vi "Build Item Graph from Type.vi"(9 "OwningVI":refnum<vi>, 10 "Max Depth (12)":i32=12, 11 "Type":variant) -> (0 "error out":errorcluster, 3 "Item Graph":T1[](array[typedef]))   [LabVIEW 2020, in "Better Search.lvlib"]
uses:
  Better Search.lvlib
  Data Types/Type Reflection Item.ctl
  <vilib>/Utility/Data Type/NI_Data Type.lvlib
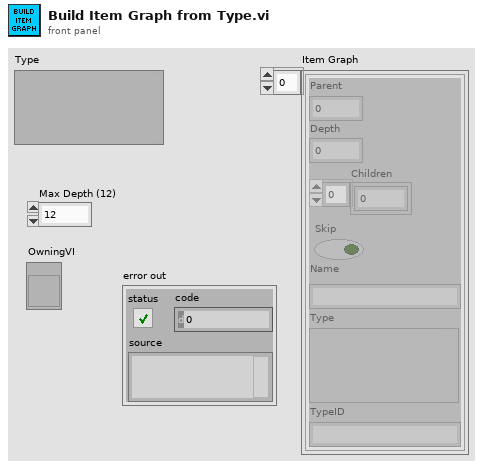
[diagram p1: front panel]
types:
  T1 = typedef "Better Search.lvlib/Type Reflection Item.ctl" = cluster{"Parent":i32, "Depth":i32, "Children":i32[], "Skip":bool, "Name":string, "Type":variant, "TypeID":string}
  T2 = typedef "NI_Data Type.lvlib/Data Type.ctl" = enum8{"Invalid Type", "Void", "I8", "I16", "I32", "I64", "U8", "U16", "U32", "U64", "Single Float", "Double Float", "Extended Float", "Single Complex", "Double Complex", "Extended Complex", "Enum U8", "Enum U16", "Enum U32", "Enum U64", "Single Float With Unit", "Double Float With Unit", "Extended Float With Unit", "Single Complex with Unit", "Double Complex with Unit", "Extended Complex with Unit", "Boolean", "String", "Path", "Picture", "Tag", "Array", "Cluster", "Variant", "LV Variant", "Waveform", "Timestamp", "Digital Waveform", "Digital Data", "ExpressData", "Refnum", "External Data", "VI", "Poly VI", "LabVIEW Class Instance", "Fixed Point", "Set Collection", "Map Collection"}
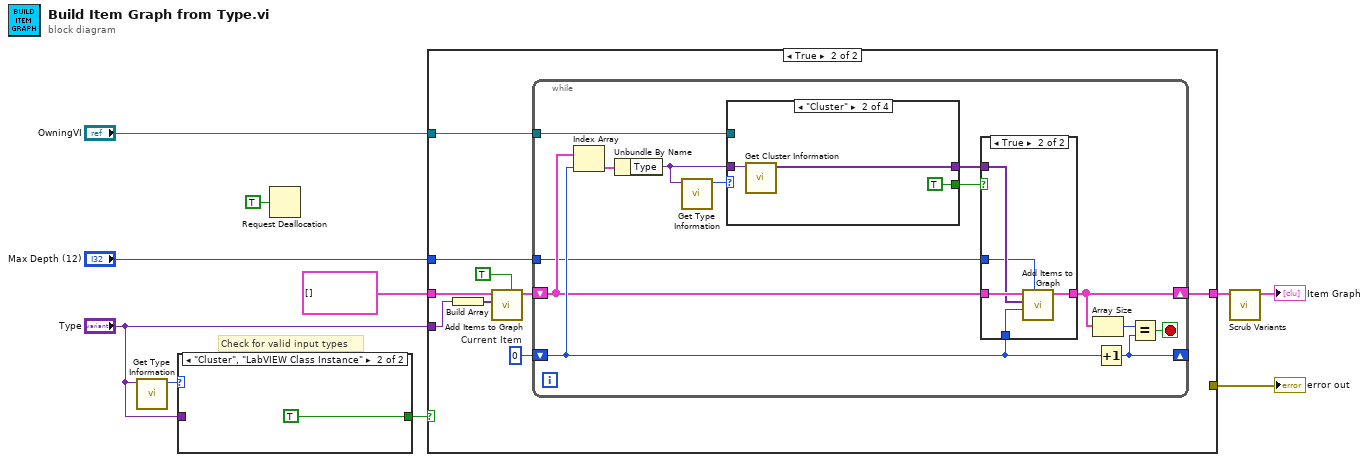
[diagram p0: block diagram]
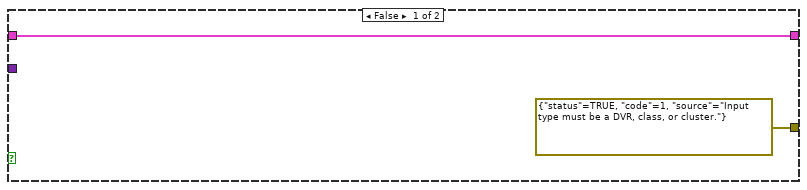
[diagram p2: hidden frame]
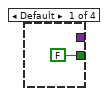
[diagram p3: hidden frame]
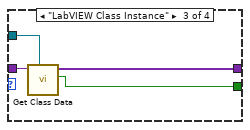
[diagram p4: hidden frame]
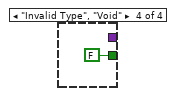
[diagram p5: hidden frame]
diagram:
  # "Check for valid input types"
  n1 = call <vilib>:"Get Type Information.vi"("variant"="Type") -> ("type"=w10:T2)  [unwired: 6 in, 4 out]
  n2 = case shown="\"Cluster\", \"LabVIEW Class Instance\"" w10 {
    tunnel: "Type" -> [_ _]
    tunnel: [_ TRUE] -> w9
    frame Default {
    }
    frame "Cluster", "LabVIEW Class Instance" {
    }
  }
  n3 = Request Deallocation(TRUE ("flag")) -> ()
  n4 = case shown="True" w9 {
    tunnel: "Type" -> [_ w20]
    tunnel: T1[] [] ("Item Graph") -> [w12 w22]
    tunnel: [w12 w18] -> w2
    tunnel: [errorcluster {"status"=TRUE, "code"=1, "source"="Input type must be a DVR, class, or cluster."} ("error constant") _] -> w6
    tunnel: "OwningVI" -> [_ w16]
    tunnel: "Max Depth (12)" -> [_ w15]
    frame False {
    }
    frame True {
      w19 = 0  # Current Item
      n5 = Build Array(w20) -> (w17:variant[])
      n6 = call "Add Items to Graph.vi"("Force Skip? (F)"=TRUE, "Items"=w17, "Graph In"=w22) -> ("Graph"=w21:T1[])  [unwired: 8 in]
      n7 = while {
        shift-right: [w32] -> w18
        shift-left: w21 -> [w30]
        shift-right: [w34] -> _
        shift-left: w19 -> [w31]
        tunnel: w16 -> [w26]
        tunnel: w15 -> [w23]
        stop <- w33 stop-if-true
        n8 = Index Array(array=w30, index=w31) -> (element=w29:T1)
        n9 = Unbundle By Name(w29) -> ("Type"=w27:variant)
        n10 = call <vilib>:"Get Type Information.vi"("variant"=w27) -> ("type"=w28:T2)  [unwired: 6 in, 4 out]
        n11 = case shown="\"Cluster\"" w28 {
          tunnel: w27 -> [_ w39 w43 _]
          tunnel: w26 -> [_ _ w42 _]
          tunnel: [FALSE TRUE w41 FALSE] -> w25
          tunnel: [_ w38 w40 _] -> w24
          frame Default {
          }
          frame "Cluster" {
            n12 = call <vilib>:"Get Cluster Information.vi"("variant"=w39) -> ("cluster elements"=w38:variant[])  [unwired: 9 in, 1 out]
          }
          frame "LabVIEW Class Instance" {
            n13 = call "Get Class Data.vi"("OwningVI"=w42, "Class"=w43) -> ("Can Access Members?"=w41:bool, "Class Data"=w40:variant[])  [unwired: 8 in]
          }
          frame "Invalid Type", "Void" {
          }
        }
        n14 = case shown="True" w25 {
          tunnel: w30 -> [w45 w50]
          tunnel: [w45 w49] -> w32
          tunnel: w31 -> [_ w48]
          tunnel: w24 -> [_ w47]
          tunnel: w23 -> [_ w46]
          frame False {
          }
          frame True {
            n15 = call "Add Items to Graph.vi"("Depth Limit (12)"=w46, "Parent Index (None)"=w48, "Items"=w47, "Graph In"=w50) -> ("Graph"=w49:T1[])  [unwired: 7 in]
          }
        }
        n16 = Array Size(array=w32) -> (size(s)=w35:i32)
        n17 = Increment(x=w31) -> (x+1=w34:i32)
        n18 = Equal?(x=w35, y=w34) -> (x = y?=w33:bool)
      }
    }
  }
  "error out" <- w6
  n19 = call "Scrub Variants.vi"("Graph In"=w2) -> ("Cleaned Graph"=→"Item Graph":T1[])  [unwired: 10 in]
